vi "publisher tests Reader 10.vi"() -> ()   [LabVIEW 2018]
uses:
  publisher action.ctl
panel:
  out "XY Graph":cluster{dbl[], dbl[]}[](graph)=[{[0.10768872290602667, 0.08453564748123094, 0.06138257205643519, 0.03822949663163945, 0.015076421206843715, -0.00807665421795202, -0.03122972964274777, -0.05438280506754349, -0.07753588049233924, -0.10068895591713499, -0.12384203134193071, -0.14699510676672645, -0.17014818219152222, -0.19330125761631795, -0.21645433304111367, -0.23960740846590944, -0.26276048389070517, -0.2859135593155009, -0.30906663474029666, -0.3322197101650924], [0.28000560522759, 0.21980440010365815, 0.15960319497972628, 0.0994019898557944, 0.03920078473186256, -0.021000420392069286, -0.08120162551600119, -0.14140283063993303, -0.20160403576386488, -0.2618052408877968, -0.32200644601172856, -0.38220765113566046, -0.44240885625959236, -0.5026100613835242, -0.562811266507456, -0.6230124716313878, -0.6832136767553197, -0.7434148818792515, -0.8036160870031835, -0.8638172921271153]}, {[0.10774138848831771, 0.08457698996332941, 0.06141259143834109, 0.03824819291335277, 0.015083794388364463, -0.008080604136623842, -0.031245002661612176, -0.05440940118660048, -0.07757379971158879, -0.10073819823657709, -0.1239025967615654, -0.1470669952865537, -0.17023139381154206, -0.19339579233653037, -0.21656019086151868, -0.23972458938650698, -0.2628889879114953, -0.2860533864364836, -0.3092177849614719, -0.3323821834864602], [0.27998534462826696, 0.21978849553318958, 0.1595916464381122, 0.0993947973430348, 0.039197948247957415, -0.020998900847119972, -0.08119574994219736, -0.14139259903727475, -0.20158944813235213, -0.2617862972274295, -0.3219831463225069, -0.3821799954175843, -0.4423768445126617, -0.5025736936077391, -0.5627705427028165, -0.6229673917978938, -0.6831642408929712, -0.7433610899880485, -0.803557939083126, -0.8637547881782035]}, {[1.0, 0.9980267284282716, 0.9921147013144779, 0.9822872507286887, 0.9685831611286311, 0.9510565162951535, 0.9297764858882513, 0.9048270524660195, 0.8763066800438636, 0.8443279255020151, 0.8090169943749475, 0.7705132427757891, 0.7289686274214116, 0.6845471059286886, 0.6374239897486896, 0.587785252292473, 0.5358267949789965, 0.48175367410171516, 0.42577929156507266, 0.36812455268467786, 0.30901699437494745, 0.24868988716485474, 0.18738131458572452, 0.12533323356430426, 0.0627905195293133, -1.6081428723391245e-16, -0.0627905195293134, -0.12533323356430437, -0.18738131458572482, -0.24868988716485485, -0.30901699437494756, -0.368124552684678, -0.4257792915650727, -0.48175367410171543, -0.5358267949789969, -0.587785252292473, -0.6374239897486897, -0.6845471059286887, -0.7289686274214117, -0.7705132427757894, -0.8090169943749473, -0.8443279255020151, -0.8763066800438636, -0.9048270524660196, -0.9297764858882515, -0.9510565162951536, -0.9685831611286311, -0.9822872507286887, -0.9921147013144779, -0.9980267284282716, -1.0, -0.9980267284282716, -0.9921147013144779, -0.9822872507286886, -0.9685831611286311, -0.9510565162951535, -0.9297764858882512, -0.9048270524660195, -0.8763066800438635, -0.844327925502015, -0.8090169943749472, -0.770513242775789, -0.7289686274214116, -0.6845471059286886, -0.6374239897486895, -0.5877852522924732, -0.5358267949789963, -0.48175367410171527, -0.42577929156507216, -0.3681245526846778, -0.30901699437494756, -0.24868988716485443, -0.18738131458572463, -0.12533323356430373, -0.06279051952931321, -1.836909530733566e-16, 0.06279051952931372, 0.12533323356430423, 0.18738131458572513, 0.24868988716485493, 0.30901699437494723, 0.36812455268467825, 0.4257792915650726, 0.4817536741017157, 0.5358267949789968, 0.5877852522924737, 0.63742398974869, 0.6845471059286886, 0.7289686274214119, 0.7705132427757894, 0.8090169943749478, 0.8443279255020153, 0.8763066800438636, 0.9048270524660197, 0.9297764858882515, 0.9510565162951538, 0.9685831611286312, 0.9822872507286887, 0.9921147013144779, 0.9980267284282716], [0.0, 0.06279051952931337, 0.12533323356430426, 0.18738131458572463, 0.2486898871648548, 0.3090169943749474, 0.368124552684678, 0.4257792915650727, 0.4817536741017153, 0.5358267949789967, 0.5877852522924731, 0.6374239897486897, 0.6845471059286887, 0.7289686274214116, 0.7705132427757893, 0.8090169943749475, 0.8443279255020151, 0.8763066800438637, 0.9048270524660196, 0.9297764858882515, 0.9510565162951535, 0.9685831611286311, 0.9822872507286887, 0.9921147013144779, 0.9980267284282716, 1.0, 0.9980267284282716, 0.9921147013144778, 0.9822872507286886, 0.9685831611286311, 0.9510565162951535, 0.9297764858882513, 0.9048270524660195, 0.8763066800438635, 0.844327925502015, 0.8090169943749475, 0.7705132427757893, 0.7289686274214114, 0.6845471059286885, 0.6374239897486895, 0.5877852522924732, 0.5358267949789967, 0.4817536741017152, 0.4257792915650725, 0.36812455268467775, 0.3090169943749471, 0.24868988716485482, 0.18738131458572457, 0.1253332335643041, 0.06279051952931314, -3.216285744678249e-16, -0.06279051952931335, -0.12533323356430429, -0.18738131458572477, -0.24868988716485502, -0.30901699437494773, -0.3681245526846783, -0.42577929156507266, -0.4817536741017154, -0.5358267949789968, -0.5877852522924734, -0.63742398974869, -0.6845471059286887, -0.7289686274214116, -0.7705132427757894, -0.8090169943749473, -0.8443279255020153, -0.8763066800438636, -0.9048270524660198, -0.9297764858882515, -0.9510565162951535, -0.9685831611286312, -0.9822872507286887, -0.9921147013144779, -0.9980267284282716, -1.0, -0.9980267284282716, -0.9921147013144779, -0.9822872507286886, -0.9685831611286311, -0.9510565162951536, -0.9297764858882512, -0.9048270524660196, -0.8763066800438634, -0.844327925502015, -0.809016994374947, -0.770513242775789, -0.7289686274214116, -0.6845471059286883, -0.6374239897486896, -0.5877852522924726, -0.5358267949789963, -0.4817536741017153, -0.4257792915650722, -0.36812455268467786, -0.3090169943749468, -0.2486898871648545, -0.18738131458572468, -0.1253332335643038, -0.06279051952931326]}, {[0.1, 0.09980267284282716, 0.0992114701314478, 0.09822872507286888, 0.09685831611286311, 0.09510565162951536, 0.09297764858882514, 0.09048270524660196, 0.08763066800438636, 0.08443279255020152, 0.08090169943749476, 0.07705132427757892, 0.07289686274214116, 0.06845471059286887, 0.06374239897486897, 0.05877852522924731, 0.05358267949789966, 0.04817536741017152, 0.042577929156507266, 0.03681245526846779, 0.030901699437494747, 0.024868988716485477, 0.018738131458572452, 0.012533323356430426, 0.006279051952931331, -1.6081428723391246e-17, -0.0062790519529313405, -0.012533323356430438, -0.018738131458572484, -0.024868988716485487, -0.030901699437494757, -0.0368124552684678, -0.04257792915650727, -0.048175367410171546, -0.05358267949789969, -0.05877852522924731, -0.06374239897486898, -0.06845471059286888, -0.07289686274214117, -0.07705132427757894, -0.08090169943749474, -0.08443279255020152, -0.08763066800438636, -0.09048270524660196, -0.09297764858882515, -0.09510565162951537, -0.09685831611286311, -0.09822872507286888, -0.0992114701314478, -0.09980267284282716, -0.1, -0.09980267284282716, -0.0992114701314478, -0.09822872507286887, -0.09685831611286311, -0.09510565162951536, -0.09297764858882512, -0.09048270524660196, -0.08763066800438635, -0.0844327925502015, -0.08090169943749473, -0.07705132427757891, -0.07289686274214116, -0.06845471059286887, -0.06374239897486896, -0.05877852522924733, -0.05358267949789963, -0.04817536741017153, -0.04257792915650722, -0.036812455268467784, -0.030901699437494757, -0.024868988716485445, -0.018738131458572463, -0.012533323356430374, -0.006279051952931321, -1.836909530733566e-17, 0.006279051952931373, 0.012533323356430424, 0.018738131458572515, 0.024868988716485494, 0.030901699437494726, 0.036812455268467825, 0.042577929156507266, 0.048175367410171574, 0.05358267949789968, 0.05877852522924737, 0.063742398974869, 0.06845471059286887, 0.07289686274214119, 0.07705132427757894, 0.08090169943749478, 0.08443279255020153, 0.08763066800438636, 0.09048270524660197, 0.09297764858882515, 0.09510565162951538, 0.09685831611286312, 0.09822872507286888, 0.0992114701314478, 0.09980267284282716], [0.0, 0.006279051952931338, 0.012533323356430426, 0.018738131458572463, 0.02486898871648548, 0.03090169943749474, 0.0368124552684678, 0.04257792915650727, 0.04817536741017153, 0.05358267949789967, 0.058778525229247314, 0.06374239897486898, 0.06845471059286888, 0.07289686274214116, 0.07705132427757894, 0.08090169943749476, 0.08443279255020152, 0.08763066800438638, 0.09048270524660196, 0.09297764858882515, 0.09510565162951536, 0.09685831611286311, 0.09822872507286888, 0.0992114701314478, 0.09980267284282716, 0.1, 0.09980267284282716, 0.09921147013144778, 0.09822872507286887, 0.09685831611286311, 0.09510565162951536, 0.09297764858882514, 0.09048270524660196, 0.08763066800438635, 0.0844327925502015, 0.08090169943749476, 0.07705132427757894, 0.07289686274214115, 0.06845471059286885, 0.06374239897486896, 0.05877852522924733, 0.05358267949789967, 0.048175367410171525, 0.04257792915650725, 0.03681245526846778, 0.030901699437494712, 0.024868988716485484, 0.01873813145857246, 0.01253332335643041, 0.0062790519529313145, -3.216285744678249e-17, -0.006279051952931335, -0.01253332335643043, -0.018738131458572477, -0.024868988716485504, -0.030901699437494774, -0.03681245526846783, -0.042577929156507266, -0.04817536741017154, -0.05358267949789968, -0.05877852522924734, -0.063742398974869, -0.06845471059286888, -0.07289686274214116, -0.07705132427757894, -0.08090169943749474, -0.08443279255020153, -0.08763066800438636, -0.09048270524660199, -0.09297764858882515, -0.09510565162951536, -0.09685831611286312, -0.09822872507286888, -0.0992114701314478, -0.09980267284282716, -0.1, -0.09980267284282716, -0.0992114701314478, -0.09822872507286887, -0.09685831611286311, -0.09510565162951537, -0.09297764858882512, -0.09048270524660196, -0.08763066800438635, -0.0844327925502015, -0.0809016994374947, -0.07705132427757891, -0.07289686274214116, -0.06845471059286883, -0.06374239897486897, -0.05877852522924726, -0.05358267949789963, -0.04817536741017153, -0.042577929156507224, -0.03681245526846779, -0.03090169943749468, -0.02486898871648545, -0.01873813145857247, -0.012533323356430379, -0.006279051952931327]}, {[0.0, 0.0, 0.0, 0.0, 0.0, 0.0, 0.0, 0.0, 0.0, 0.0, 0.0, 0.0, 0.0, 0.0, 0.0, 0.0, 0.0, 0.0, 0.0, 0.0], [1.1, 1.135, 1.1700000000000002, 1.205, 1.24, 1.2750000000000001, 1.31, 1.345, 1.3800000000000001, 1.415, 1.4500000000000002, 1.485, 1.52, 1.5550000000000002, 1.59, 1.625, 1.6600000000000001, 1.695, 1.73, 1.7650000000000001]}, {[0.918181493751524, 0.9265285982401742, 0.9348757027288245, 0.9432228072174746, 0.9515699117061248, 0.9599170161947751, 0.9682641206834253, 0.9766112251720754, 0.9849583296607257, 0.9933054341493759, 1.0016525386380262, 1.0099996431266762, 1.0183467476153265, 1.0266938521039768, 1.0350409565926268, 1.0433880610812771, 1.0517351655699274, 1.0600822700585775, 1.0684293745472278, 1.076776479035878], [0.6057579917196472, 0.6112648825534621, 0.6167717733872771, 0.6222786642210921, 0.6277855550549071, 0.633292445888722, 0.6387993367225371, 0.644306227556352, 0.649813118390167, 0.6553200092239819, 0.6608269000577969, 0.6663337908916119, 0.6718406817254269, 0.6773475725592418, 0.6828544633930569, 0.6883613542268718, 0.6938682450606868, 0.6993751358945017, 0.7048820267283167, 0.7103889175621317]}, {[-0.7402719588478437, -0.7470017039282786, -0.7537314490087136, -0.7604611940891485, -0.7671909391695835, -0.7739206842500184, -0.7806504293304534, -0.7873801744108883, -0.7941099194913233, -0.8008396645717581, -0.807569409652193, -0.814299154732628, -0.821028899813063, -0.8277586448934979, -0.8344883899739328, -0.8412181350543678, -0.8479478801348027, -0.8546776252152377, -0.8614073702956726, -0.8681371153761075], [-0.8136322430579903, -0.8210288998130629, -0.8284255565681355, -0.8358222133232083, -0.8432188700782809, -0.8506155268333535, -0.8580121835884261, -0.8654088403434987, -0.8728054970985715, -0.8802021538536441, -0.8875988106087167, -0.8949954673637893, -0.9023921241188619, -0.9097887808739347, -0.9171854376290073, -0.9245820943840799, -0.9319787511391525, -0.9393754078942251, -0.9467720646492979, -0.9541687214043705]}]
  out "number":dbl
  in  "read":bool
  out "Numeric":i32
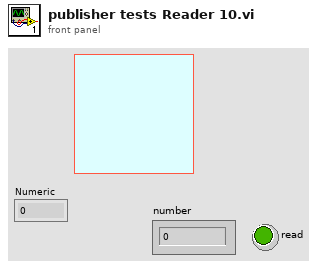
[diagram p1: front panel]
types:
  T1 = typedef "publisher action.ctl" = enum16{"set", "get", "init", "check"}
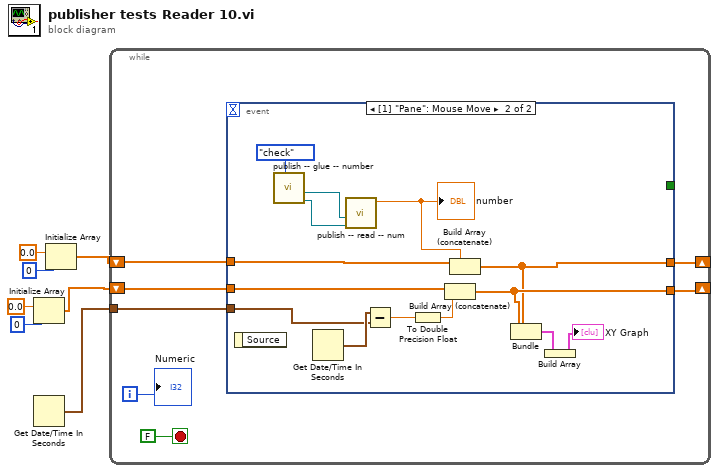
[diagram p0: block diagram]
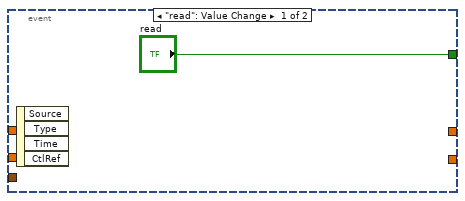
[diagram p2: hidden frame]
diagram:
  n1 = Initialize Array(0.0 ("element"), 0 ("dimension size")) -> (w1:dbl[])
  n2 = Get Date/Time In Seconds() -> (seconds since 1Jan1904=w7:timestamp)
  n3 = Initialize Array(0.0 ("element"), 0 ("dimension size")) -> (w6:dbl[])
  n4 = while {
    shift-right: [w12] -> _
    shift-left: w6 -> [w11]
    tunnel: w7 -> [w10]
    shift-right: [w9] -> _
    shift-left: w1 -> [w8]
    i -> [w13]
    stop <- FALSE stop-if-true
    n5 = event shown="[1] \"Pane\": Mouse Move" {
      selector: _ -> [_ _]
      dyn-events: _ -> [_ _]
      timeout: _ -> [_ _]
      tunnel: ["read" _] -> _
      tunnel: [_ w18] -> w12
      tunnel: w11 -> [_ w25]
      tunnel: w10 -> [_ w22]
      tunnel: [_ w19] -> w9
      tunnel: w8 -> [_ w20]
      event "read": Value Change {
        n6 = event-data() -> ()  [unwired: 1 in, 4 out]
      }
      event Mouse Move {
        n7 = event-data() -> ()  [unwired: 1 in, 1 out]
        n8 = call "publish -- glue -- number.vi"("publisher action"=publisher_action."check") -> ("request event"=w28:refnum<user-event>, "response out"=w27:refnum<user-event>)  [unwired: 8 in, 1 out]
        n9 = Get Date/Time In Seconds() -> (seconds since 1Jan1904=w24:timestamp)
        n10 = call "publish -- read -- num.vi"("request event"=w28, "response in"=w27) -> ("Numeric"=w26:dbl)  [unwired: 8 in, 1 out]
        "number" <- w26
        n11 = Subtract(x=w24, y=w22) -> (x-y=w23:dbl)
        n12 = To Double Precision Float(number=w23) -> (double precision float=w21:dbl)
        n13 = Build Array (concatenate)(w20, w21) -> (w19:dbl[])
        n14 = Build Array (concatenate)(w25, w26) -> (w18:dbl[])
        n15 = Bundle(w19, w18) -> (w17:cluster{dbl[], dbl[]})  [unwired: 1 in]
        n16 = Build Array(w17) -> (→"XY Graph":cluster{dbl[], dbl[]}[])
      }
    }
    "Numeric" <- w13
  }
